vi "Pretty Print 2.vi"(0 "JSON String":string) -> (1 "Invalid JSON":bool, 2 "Pretty JSON String":string)   [LabVIEW 2011, in "LV JSON.lvlib"]
doc: "Format JSON string with white space to make it readable.\n\nInvalid JSON boolean indicates when the input JSON string is missing a close bracket or close brace. (It does NOT check for valid JSON formatting.)"
uses:
  LV JSON.lvlib
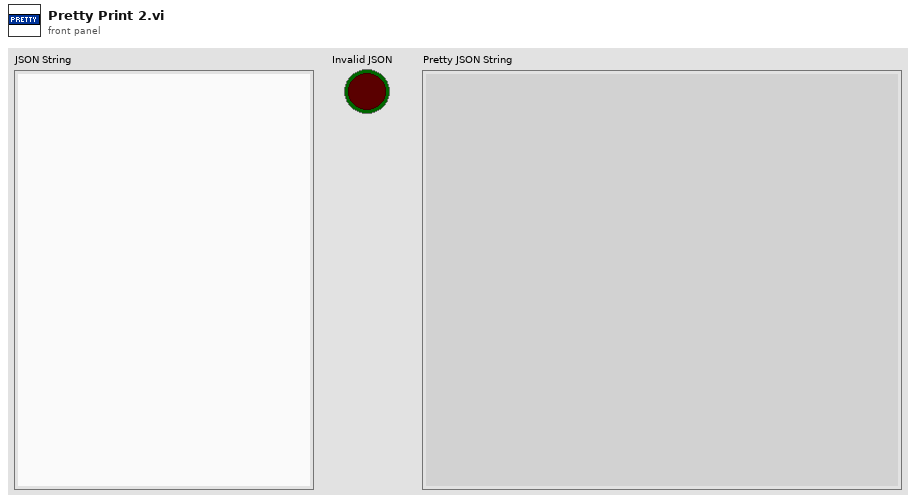
[diagram p1: front panel]
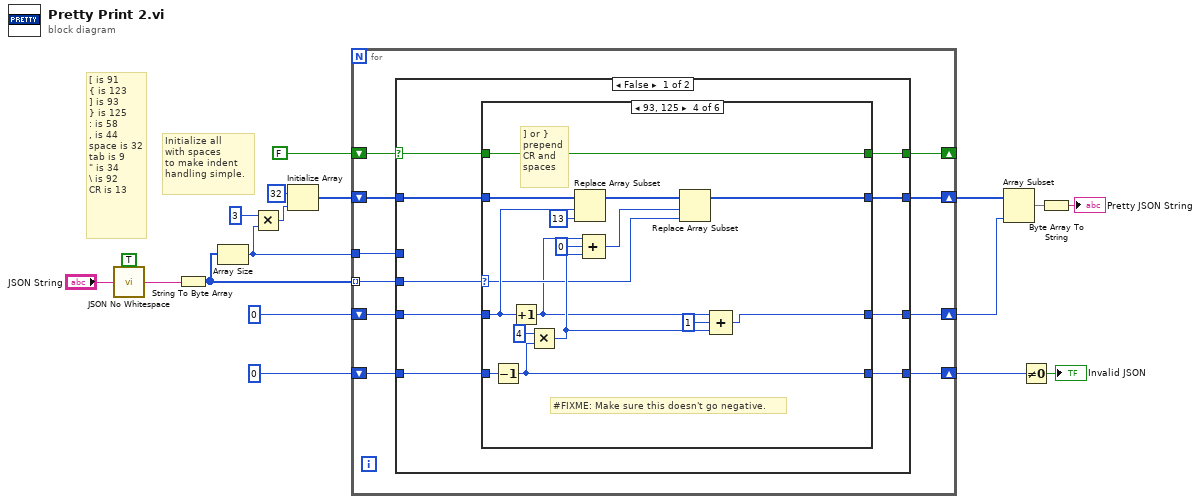
[diagram p0: block diagram]
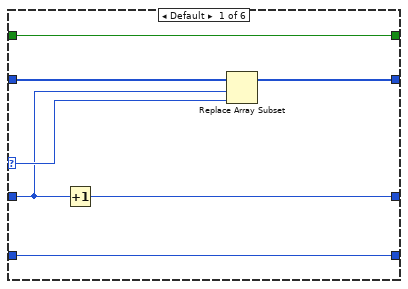
[diagram p2: hidden frame]
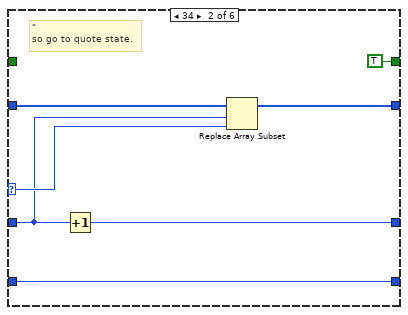
[diagram p3: hidden frame]
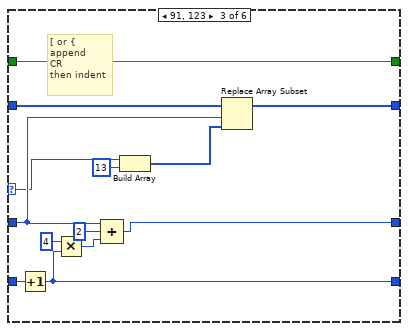
[diagram p4: hidden frame]
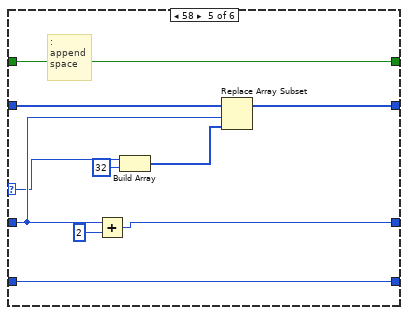
[diagram p5: hidden frame]
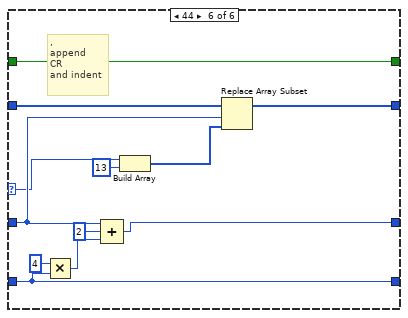
[diagram p6: hidden frame]
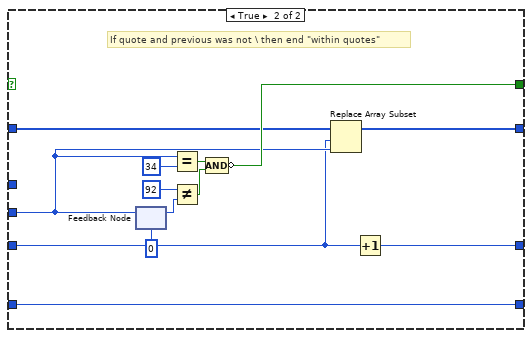
[diagram p7: hidden frame]
diagram:
  # "Initialize all\nwith spaces\nto make indent\nhandling simple."
  # "[ is 91\n{ is 123\n] is 93\n} is 125\n: is 58\n, is 44\nspace is 32\ntab is 9\n\" is 34\n\\ is 92\nCR is 13"
  n1 = call "JSON No Whitespace.vi"("String"="JSON String", "Except in Quotes (F)"=TRUE) -> ("Trimmed String"=w15:string)
  n2 = String To Byte Array(string=w15) -> (unsigned byte array=w11:u8[])
  n3 = Array Size(array=w11) -> (size(s)=w10:i32)
  n4 = Multiply(x=3, y=w10) -> (x*y=w13:i32)
  n5 = Initialize Array(u8 32, w13) -> (w12:u8[])
  n6 = for {
    shift-right: [w22] -> w6
    shift-left: w12 -> [w19]
    tunnel: w11 -> [w25] mode=indexing
    shift-right: [w27] -> _
    shift-left: FALSE -> [w28]
    tunnel: w10 -> [w26]
    shift-right: [w23] -> w5
    shift-left: 0 -> [w24]
    shift-right: [w20] -> w3
    shift-left: 0 -> [w21]
    n7 = case shown="False" w28 {
      selector: w28 -> [w30 _]
      tunnel: [w29 w109] -> w27
      tunnel: w19 -> [w36 w106]
      tunnel: w26 -> [_ _]
      tunnel: w25 -> [w37 w104]
      tunnel: w24 -> [w35 w103]
      tunnel: [w34 w107] -> w23
      tunnel: [w33 w105] -> w22
      tunnel: w21 -> [w32 w108]
      tunnel: [w31 w108] -> w20
      frame False {
        n8 = case shown="93, 125" w37 {
          selector: w37 -> [w41 w49 w60 w66 w86 w98]
          tunnel: w36 -> [w43 w51 w64 w80 w90 w102]
          tunnel: w35 -> [w40 w48 w61 w69 w87 w99]
          tunnel: [w39 w47 w63 w79 w89 w101] -> w34
          tunnel: [w42 w50 w57 w71 w83 w95] -> w33
          tunnel: w32 -> [w38 w46 w56 w77 w81 w92]
          tunnel: [w38 w46 w53 w75 w81 w92] -> w31
          tunnel: w30 -> [w44 _ w52 w74 w82 w94]
          tunnel: [w44 TRUE w52 w74 w82 w94] -> w29
          frame Default {
            n9 = Increment(x=w40) -> (x+1=w39:i32)
            n10 = Replace Array Subset(array=w43, new element=w41, index=w40) -> (w42:u8[])
          }
          frame 34 {
            # "\"\nso go to quote state."
            n11 = Increment(x=w48) -> (x+1=w47:i32)
            n12 = Replace Array Subset(array=w51, new element=w49, index=w48) -> (w50:u8[])
          }
          frame 91, 123 {
            # "[ or {\nappend\nCR\nthen indent"
            n13 = Increment(x=w56) -> (x+1=w53:i32)
            n14 = Multiply(x=4 ("y"), y=w53) -> (x*y=w54:i32)
            n15 = Compound Arithmetic op=ADD(w61, 2 ("y"), w54) -> (w63:i32)
            n16 = Build Array(w60, u8 13 ("element")) -> (w59:u8[])
            n17 = Replace Array Subset(array=w64, new element=w59, index=w61) -> (w57:u8[])
          }
          frame 93, 125 {
            # "#FIXME: Make sure this doesn't go negative."
            # "] or }\nprepend\nCR and\nspaces"
            n18 = Decrement(x=w77) -> (x-1=w75:i32)
            n19 = Increment(x=w69) -> (x+1=w65:i32)
            n20 = Multiply(x=4 ("y"), y=w75) -> (x*y=w68:i32)
            n21 = Replace Array Subset(array=w80, new element=u8 13 ("element"), index=w69) -> (w72:u8[])
            n22 = Compound Arithmetic op=ADD(w65, 0 ("y"), w68) -> (w67:i32)
            n23 = Replace Array Subset(array=w72, new element=w66, index=w67) -> (w71:u8[])
            n24 = Compound Arithmetic op=ADD(w65, 1 ("y"), w68) -> (w79:i32)
          }
          frame 58 {
            # ":\nappend\nspace"
            n25 = Add(x=w87, y=2) -> (x+y=w89:i32)
            n26 = Build Array(w86, u8 32 ("element")) -> (w85:u8[])
            n27 = Replace Array Subset(array=w90, new element=w85, index=w87) -> (w83:u8[])
          }
          frame 44 {
            # ",\nappend\nCR\nand indent"
            n28 = Multiply(x=4 ("y"), y=w92) -> (x*y=w91:i32)
            n29 = Compound Arithmetic op=ADD(w99, 2 ("y"), w91) -> (w101:i32)
            n30 = Build Array(w98, u8 13 ("element")) -> (w97:u8[])
            n31 = Replace Array Subset(array=w102, new element=w97, index=w99) -> (w95:u8[])
          }
        }
      }
      frame True {
        # "If quote and previous was not \\ then end \"within quotes\""
        n32 = feedback #1(u8 0 ("x")) -> (w112:u8)
        n33 = feedback-in #1(w104) -> ()
        n34 = Equal?(x=w104, y=u8 34) -> (x = y?=w114:bool)
        n35 = Not Equal?(x=u8 92, y=w112) -> (x != y?=w115:bool)
        n36 = Compound Arithmetic op=AND(w114, w115) -> (invert w109:bool)
        n37 = Replace Array Subset(array=w106, new element=w104, index=w103) -> (w105:u8[])
        n38 = Increment(x=w103) -> (x+1=w107:i32)
      }
    }
  }
  n39 = Array Subset(array=w6, length=w5) -> (w4:u8[])  [unwired: 1 in]
  n40 = Not Equal To 0?(x=w3) -> (x != 0?=→"Invalid JSON":bool)
  n41 = Byte Array To String(unsigned byte array=w4) -> (string=→"Pretty JSON String":string)
